vi "test_PhotonPoseEstimator_ClosestToRefPose.vi"(8 "error in (no error)":errorcluster) -> (0 "error out":errorcluster, 3 "Test Passed":bool)   [LabVIEW 2019]
uses:
  <vilib>/Rock Robotics/WPI/ThirdParty/PhotonVisionLib/TypeDef/PhotonEstimatedRobotPoseType.ctl
  <vilib>/Rock Robotics/WPI/ThirdParty/JAS_Junk/TrajLib/TypeDef/POSE3D.ctl
  <vilib>/Rock Robotics/WPI/ThirdParty/JAS_Junk/TrajLib/TypeDef/TRANSLATION3D.ctl
  <vilib>/Rock Robotics/WPI/ThirdParty/JAS_Junk/TrajLib/TypeDef/ROTATION3D.ctl
  <vilib>/Rock Robotics/WPI/ThirdParty/JAS_Junk/TrajLib/TypeDef/QUATERNION.ctl
  <vilib>/Rock Robotics/WPI/ThirdParty/PhotonVisionLib/TypeDef/PhotonTrackedTargetType.ctl
  <vilib>/Rock Robotics/WPI/ThirdParty/PhotonVisionLib/TypeDef/TargetCornerType.ctl
  <vilib>/Rock Robotics/WPI/ThirdParty/JAS_Junk/TrajLib/TypeDef/TRANSFORM3D.ctl
  <vilib>/Rock Robotics/WPI/ThirdParty/PhotonPoseStrategy_ENUM.ctl
  <vilib>/Rock Robotics/WPI/ThirdParty/JAS_Junk/TrajLib/VI/Quaternion_New.vi
  <vilib>/Rock Robotics/WPI/ThirdParty/PhotonVisionLib/SubVI/PhotonTargetModel_New_AprilTag16h5.vi
  <vilib>/Rock Robotics/WPI/ThirdParty/PhotonVisionLib/SubVI/PhotonPoseEstimator_Update_All.vi
  <vilib>/Rock Robotics/WPI/ThirdParty/PhotonVisionLib/SubVI/PhotonTargetModel_New_RectPlanar.vi
  <vilib>/Rock Robotics/WPI/ThirdParty/JAS_Junk/TrajLib/Conv_Inches_Meters.vi
  <vilib>/Rock Robotics/WPI/ThirdParty/PhotonVisionLib/SubVI/PhotonPoseEstimator_SetLastPose.vi
  <vilib>/Rock Robotics/WPI/ThirdParty/PhotonVisionLib/SubVI/PhotonPoseEstimator_GetEmptyPose.vi
  <vilib>/Rock Robotics/WPI/ThirdParty/PhotonVisionLib/SubVI/PhotonPoseEstimator_lowestAmbiguityStrategy.vi
  <vilib>/Rock Robotics/WPI/ThirdParty/PhotonVisionLib/SubVI/PhotonPoseEstimator_closestToCameraHeightStrategy.vi
  <vilib>/Rock Robotics/WPI/ThirdParty/PhotonVisionLib/SubVI/PhotonPoseEstimator_closestToReferencePoseStrategy.vi
  <vilib>/Rock Robotics/WPI/ThirdParty/PhotonVisionLib/SubVI/PhotonPoseEstimator_GetReferencePose.vi
  <vilib>/Rock Robotics/WPI/ThirdParty/PhotonVisionLib/SubVI/PhotonPoseEstimator_GetLastPose.vi
  <vilib>/Rock Robotics/WPI/ThirdParty/PhotonVisionLib/SubVI/PhotonPoseEstimator_averageBestTargetsStrategy.vi
  <vilib>/Rock Robotics/WPI/ThirdParty/PhotonVisionLib/SubVI/PhotonPoseEstimator_multiTagOnCoprocStrategy.vi
  <vilib>/Rock Robotics/WPI/ThirdParty/PhotonVisionLib/SubVI/PhotonTargetModel_New.vi
  <vilib>/Rock Robotics/WPI/ThirdParty/JAS_Junk/TrajLib/VI/Rotation3d_Create_AxisAngle.vi
  <vilib>/Rock Robotics/WPI/ThirdParty/JAS_Junk/TrajLib/VI/Pose3d_New.vi
  <vilib>/Rock Robotics/WPI/ThirdParty/PhotonVisionLib/SubVI/PhotonPipelineResult_HasTargets.vi
  <vilib>/Rock Robotics/WPI/ThirdParty/PhotonVisionLib/SubVI/PhotonPipelineResult_GetTargets.vi
  <vilib>/Rock Robotics/WPI/ThirdParty/PhotonVisionLib/SubVI/PhotonTrackedTarget_GetPoseAmbiguity.vi
  <vilib>/Rock Robotics/WPI/ThirdParty/PhotonVisionLib/SubVI/PhotonTrackedTarget_GetFiducialId.vi
  <vilib>/Rock Robotics/WPI/ThirdParty/PhotonVisionLib/SubVI/PhotonPoseEstimator_GetFieldTags.vi
  <vilib>/Rock Robotics/WPI/ThirdParty/JAS_Junk/TrajLib/VI/AprilTagFieldLayout_GetTagPose.vi
  <vilib>/Rock Robotics/WPI/ThirdParty/JAS_Junk/TrajLib/VI/Pose3d_TransformBy.vi
  <vilib>/Rock Robotics/WPI/ThirdParty/PhotonVisionLib/SubVI/PhotonTrackedTarget_GetBestCameraToTarget.vi
  <vilib>/Rock Robotics/WPI/ThirdParty/JAS_Junk/TrajLib/VI/Transform3d_Inverse.vi
  <vilib>/Rock Robotics/WPI/ThirdParty/PhotonVisionLib/SubVI/PhotonPoseEstimator_GetHighestAmbiguity.vi
  <vilib>/Rock Robotics/WPI/ThirdParty/PhotonVisionLib/SubVI/PhotonPipelineResult_GetTimeStampSecs.vi
  <vilib>/Rock Robotics/WPI/ThirdParty/PhotonVisionLib/SubVI/PhotonPoseEstimator_GetRobotToCameraTransform.vi
  <vilib>/Rock Robotics/WPI/ThirdParty/PhotonVisionLib/SubVI/PhotonEstimatedRobotPose_New.vi
  <vilib>/Rock Robotics/WPI/ThirdParty/PhotonVisionLib/SubVI/PhotonPoseEstimator_closestToCameraHeightStrategy_calc.vi
  <vilib>/Rock Robotics/WPI/ThirdParty/PhotonVisionLib/SubVI/PhotonTrackedTarget_GetAltCameraToTarget.vi
  <vilib>/Rock Robotics/WPI/ThirdParty/PhotonVisionLib/SubVI/PhotonPoseEstimator_closestToReferencePoseStrategy_calc.vi
  <vilib>/Rock Robotics/WPI/ThirdParty/PhotonVisionLib/SubVI/PhotonPoseEstimator_averageBestTargetsStrategy_calc.vi
  <vilib>/Rock Robotics/WPI/ThirdParty/JAS_Junk/TrajLib/VI/Rotation3d_Plus.vi
  <vilib>/Rock Robotics/WPI/ThirdParty/JAS_Junk/TrajLib/VI/Translation3d_Plus.vi
  <vilib>/Rock Robotics/WPI/ThirdParty/JAS_Junk/TrajLib/VI/Translation3d_Times.vi
  <vilib>/Rock Robotics/WPI/ThirdParty/JAS_Junk/TrajLib/VI/Rotation3d_Times.vi
  <vilib>/Rock Robotics/WPI/ThirdParty/JAS_Junk/TrajLib/VI/Rotation3d_Create_Default.vi
  <vilib>/Rock Robotics/WPI/ThirdParty/JAS_Junk/TrajLib/VI/Translation3d_Create_Default.vi
  <vilib>/Rock Robotics/WPI/ThirdParty/JAS_Junk/TrajLib/VI/Pose3d_New_Default.vi
  <vilib>/Rock Robotics/WPI/ThirdParty/JAS_Junk/TrajLib/VI/Pose3d_Plus.vi
  <vilib>/Rock Robotics/WPI/ThirdParty/JAS_Junk/TrajLib/VI/Pose3d_RelativeTo.vi
  <vilib>/Rock Robotics/WPI/ThirdParty/JAS_Junk/TrajLib/VI/AprilTagFieldLayout_GetOriginPosition.vi
  <vilib>/Rock Robotics/WPI/ThirdParty/PhotonVisionLib/SubVI/PhotonPipelineResult_GetMultiTagResult.vi
  <vilib>/Rock Robotics/WPI/ThirdParty/JAS_Junk/TrajLib/VI/Vector_Norm.vi
  <vilib>/Rock Robotics/WPI/ThirdParty/JAS_Junk/TrajLib/VecBuilder_ArrayBy1Fill.vi
  <vilib>/Rock Robotics/WPI/ThirdParty/JAS_Junk/TrajLib/VI/AprilTag_GetAll.vi
  <vilib>/Rock Robotics/WPI/ThirdParty/JAS_Junk/TrajLib/VI/Pose3d_getTranslation3d.vi
  <vilib>/Rock Robotics/WPI/ThirdParty/JAS_Junk/TrajLib/VI/Pose3d_getRotation3d.vi
  <vilib>/Rock Robotics/WPI/ThirdParty/JAS_Junk/TrajLib/VI/Transform3d_GetTranslation3d.vi
  <vilib>/Rock Robotics/WPI/ThirdParty/JAS_Junk/TrajLib/VI/Transform3d_GetRotation3d.vi
  <vilib>/Rock Robotics/WPI/ThirdParty/JAS_Junk/TrajLib/VI/Translation3d_RotateBy.vi
  <vilib>/Rock Robotics/WPI/ThirdParty/JAS_Junk/TrajLib/VI/Translation3d_ToTranslation2d.vi
  <vilib>/Rock Robotics/WPI/ThirdParty/JAS_Junk/TrajLib/VI/Rotation3d_ToRotation2d.vi
  <vilib>/Rock Robotics/WPI/ThirdParty/JAS_Junk/TrajLib/Transform2d_Create_TransRot.vi
  <vilib>/Rock Robotics/WPI/ThirdParty/JAS_Junk/TrajLib/VI/Rotation3d_UnaryMinus.vi
  <vilib>/Rock Robotics/WPI/ThirdParty/JAS_Junk/TrajLib/VI/Translation3d_UnaryMinus.vi
  <vilib>/Rock Robotics/WPI/ThirdParty/JAS_Junk/TrajLib/VI/Transform3d_GetXYZ.vi
  <vilib>/Rock Robotics/WPI/ThirdParty/JAS_Junk/TrajLib/VI/Pose3d_getXYZ.vi
  <vilib>/Rock Robotics/WPI/ThirdParty/PhotonVisionLib/SubVI/PhotonPoseEstimator_CalcDifference.vi
  <vilib>/Rock Robotics/WPI/ThirdParty/JAS_Junk/TrajLib/VI/Rotation3d_RotateBy.vi
  <vilib>/Rock Robotics/WPI/ThirdParty/JAS_Junk/TrajLib/VI/Translation3d_GetXYZ.vi
  <vilib>/Rock Robotics/WPI/ThirdParty/JAS_Junk/TrajLib/VI/Rotation3d_GetQuaterion.vi
  <vilib>/Rock Robotics/WPI/ThirdParty/JAS_Junk/TrajLib/VI/Quaternion_Get_Vect.vi
  <vilib>/Rock Robotics/WPI/ThirdParty/JAS_Junk/TrajLib/VI/Quaternion_Get_W.vi
  <vilib>/Rock Robotics/WPI/ThirdParty/JAS_Junk/TrajLib/VI/Quaternion_New_Default.vi
  <vilib>/Rock Robotics/WPI/ThirdParty/JAS_Junk/TrajLib/VI/Transform3d_Create_Pose3dPose3d.vi
  <vilib>/Rock Robotics/WPI/ThirdParty/JAS_Junk/TrajLib/MatBuilder_Create.vi
  <vilib>/Rock Robotics/WPI/ThirdParty/JAS_Junk/TrajLib/VI/Quaternion_Times.vi
  <vilib>/Rock Robotics/WPI/ThirdParty/JAS_Junk/TrajLib/VI/Quaternion_Inverse.vi
  <vilib>/Rock Robotics/WPI/ThirdParty/JAS_Junk/TrajLib/VI/Quaternion_Get_All.vi
  <vilib>/Rock Robotics/WPI/ThirdParty/JAS_Junk/TrajLib/Translation2d_Create.vi
  <vilib>/Rock Robotics/WPI/ThirdParty/JAS_Junk/TrajLib/Rotation2d_CreateAngle.vi
  <vilib>/Rock Robotics/WPI/ThirdParty/JAS_Junk/TrajLib/VI/Rotation3d_GetXYZ.vi
  <vilib>/Rock Robotics/WPI/ThirdParty/JAS_Junk/TrajLib/VI/Rotation3d_Create_Quaternion.vi
  <vilib>/Rock Robotics/WPI/ThirdParty/JAS_Junk/TrajLib/VI/Translation3d_GetDistance.vi
  <vilib>/Rock Robotics/WPI/ThirdParty/JAS_Junk/TrajLib/VI/Translation3d_Minus.vi
  <vilib>/Rock Robotics/WPI/ThirdParty/JAS_Junk/TrajLib/VI/Rotation3d_Minus.vi
  <vilib>/Rock Robotics/WPI/ThirdParty/JAS_Junk/TrajLib/VI/Quaternion_Normalize.vi
  <vilib>/Rock Robotics/WPI/ThirdParty/PhotonVisionLib/SubVI/PhotonCamera_GetDistCoeffs.vi
  <vilib>/Rock Robotics/WPI/ThirdParty/PhotonVisionLib/SubVI/PhotonCamera_GetCameraMatrix.vi
  <vilib>/Rock Robotics/WPI/ThirdParty/JAS_Junk/TrajLib/Trajectory_Library.lvlib
  <vilib>/Rock Robotics/WPI/ThirdParty/PhotonVisionLib/PhotonVisionLib.lvlib
panel:
  out "Pos Found":bool
  out "PhotonEstimatedRobotPose":T1={"EstimatedPose"={"Translation3d"={"X"=0.0, "Y"=0.0, "Z"=0.0}, "Rotation3d"={"Q_quaternion"={"R"=1.0, "V"=[0.0, 0.0, 0.0]}}}, "TimeStamp_Seconds"=0.0, "targetsUsed"=[], "Strategy"=enum."LOWEST_AMBIGUITY"} {"targetsUsed"."AltCameraToTarget"."TRANSLATION3D"."Z" format="%14.3f"; "targetsUsed"."AltCameraToTarget"."TRANSLATION3D"."Y" format="%14.3f"; "targetsUsed"."AltCameraToTarget"."TRANSLATION3D"."X" format="%14.3f"; "targetsUsed"."BestCameraToTarget"."TRANSLATION3D"."Z" format="%14.3f"; "targetsUsed"."BestCameraToTarget"."TRANSLATION3D"."Y" format="%14.3f"; "targetsUsed"."BestCameraToTarget"."TRANSLATION3D"."X" format="%14.3f"; "EstimatedPose"."Translation3d"."Z" format="%14.3f"; "EstimatedPose"."Translation3d"."Y" format="%14.3f"; "EstimatedPose"."Translation3d"."X" format="%14.3f"}
  out "Test 0 Passed":bool
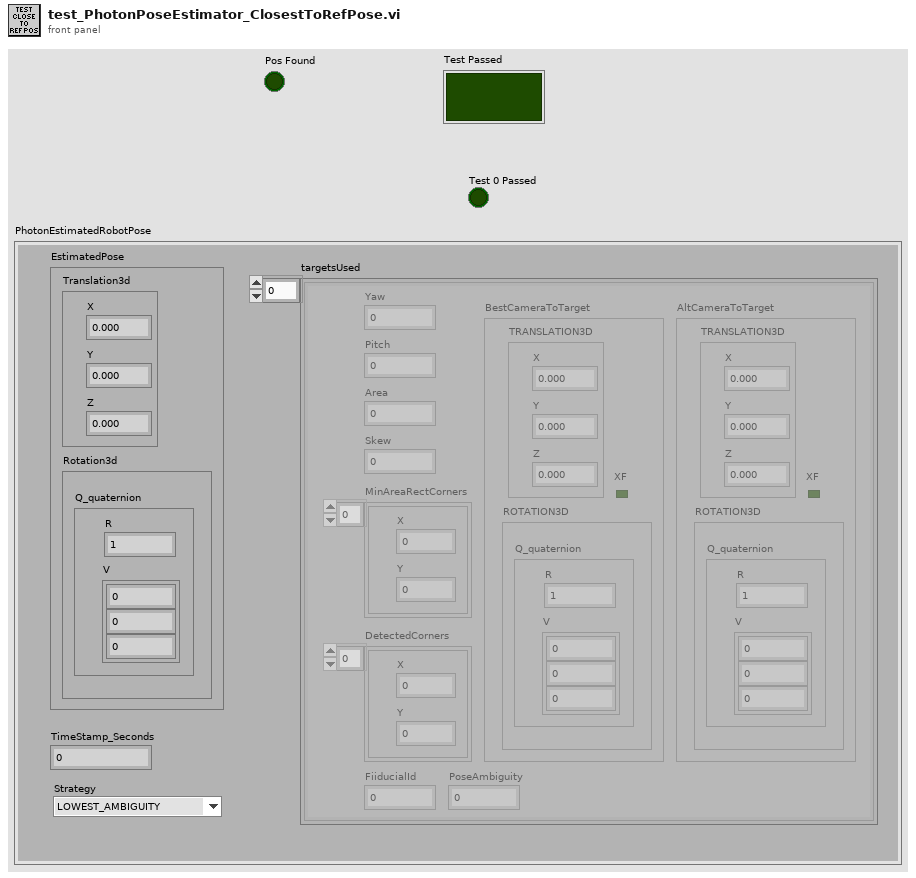
[diagram p1: front panel]
types:
  T1 = typedef "PhotonVisionLib.lvlib/PhotonEstimatedRobotPoseType.ctl" = cluster{"EstimatedPose":T2, "TimeStamp_Seconds":dbl, "targetsUsed":T6[], "Strategy":T9}
  T2 = typedef "Trajectory_Library.lvlib/POSE3D.ctl" = cluster{"Translation3d":T3, "Rotation3d":T4}
  T3 = typedef "Trajectory_Library.lvlib/TRANSLATION3D.ctl" = cluster{"X":dbl, "Y":dbl, "Z":dbl}
  T4 = typedef "Trajectory_Library.lvlib/ROTATION3D.ctl" = cluster{"Q_quaternion":T5}
  T5 = typedef "Trajectory_Library.lvlib/QUATERNION.ctl" = cluster{"R":dbl, "V":dbl[]}
  T6 = typedef "PhotonVisionLib.lvlib/PhotonTrackedTargetType.ctl" = cluster{"Yaw":dbl, "Pitch":dbl, "Area":dbl, "Skew":dbl, "MinAreaRectCorners":T7[], "BestCameraToTarget":T8, "FiiducialId":i32, "AltCameraToTarget":T8, "PoseAmbiguity":dbl, "DetectedCorners":T7[]}
  T7 = typedef "PhotonVisionLib.lvlib/TargetCornerType.ctl" = cluster{"X":dbl, "Y":dbl}
  T8 = typedef "Trajectory_Library.lvlib/TRANSFORM3D.ctl" = cluster{"TRANSLATION3D":T3, "ROTATION3D":T4, "XF":bool}
  T9 = typedef "PhotonVisionLib.lvlib/PhotonPoseStrategy_ENUM.ctl" = enum16{"LOWEST_AMBIGUITY", "CLOSEST_TO_CAMERA_HEIGHT", "CLOSEST_TO_REFERENCE_POSE", "CLOSEST_TO_LAST_POSE", "AVERAGE_BEST_TARGETS", "MULTI_TAG_PNP_ON_COPROCESSOR", "MULTI_TAG_PNP_ON_RIO"}
  T10 = typedef "Trajectory_Library.lvlib/AprilTagFieldLayout.ctl" = cluster{"AprilTagMap":map{i32, T11}, "FieldLength":dbl, "FieldWidth":dbl, "OriginPosition ":T12, "OriginPose3d":T2}
  T11 = typedef "Trajectory_Library.lvlib/AprilTag.ctl" = cluster{"ID":i32, "POSE3D":T2}
  T12 = typedef "Trajectory_Library.lvlib/AprilTagFieldLayoutOrignPosition_ENUM.ctl" = enum16{"kBlueAllianceWallRightSide,", "kRedAllianceWallRightSide,"}
  T13 = typedef "PhotonVisionLib.lvlib/PhotonPipelineResultType.ctl" = cluster{"TargetCount":i32, "Latency_MilliSec":dbl, "Targets":T6[], "TimeStampSec":dbl, "PhotonMultiTargetPNPResult":T14}
  T14 = typedef "PhotonVisionLib.lvlib/PhotonMultiTargetPNPResultType.ctl" = cluster{"PhotonPNPResult":T15, "FiducialIDsUsed":i16[]}
  T15 = typedef "PhotonVisionLib.lvlib/PhotonPNPResultType.ctl" = cluster{"IsPresent":bool, "bestReprojErr":dbl, "altReprojErr":dbl, "ambiguity":dbl, "Best":T8, "Alt":T8}
  T16 = typedef "PhotonVisionLib.lvlib/PhotonPoseEstimatorType.ctl" = cluster{"LastPose":T2, "ReferencePose":T2, "FieldTags":T10, "PrimaryStratety":T9, "Camera":string, "RobotToCamera":T8, "ReportedErrors":dbl[], "HighestAmbiguity":dbl, "MultiTagFallbackStrategy":T9, "PoseCacheTimeoutSec":dbl, "PhotonTargetModel":T17, "BaseNTName":string}
  T17 = typedef "PhotonVisionLib.lvlib/PhotonTargetModel.ctl" = cluster{"Vertices":T3[], "IsPlaner":bool, "IsSpherical":bool}
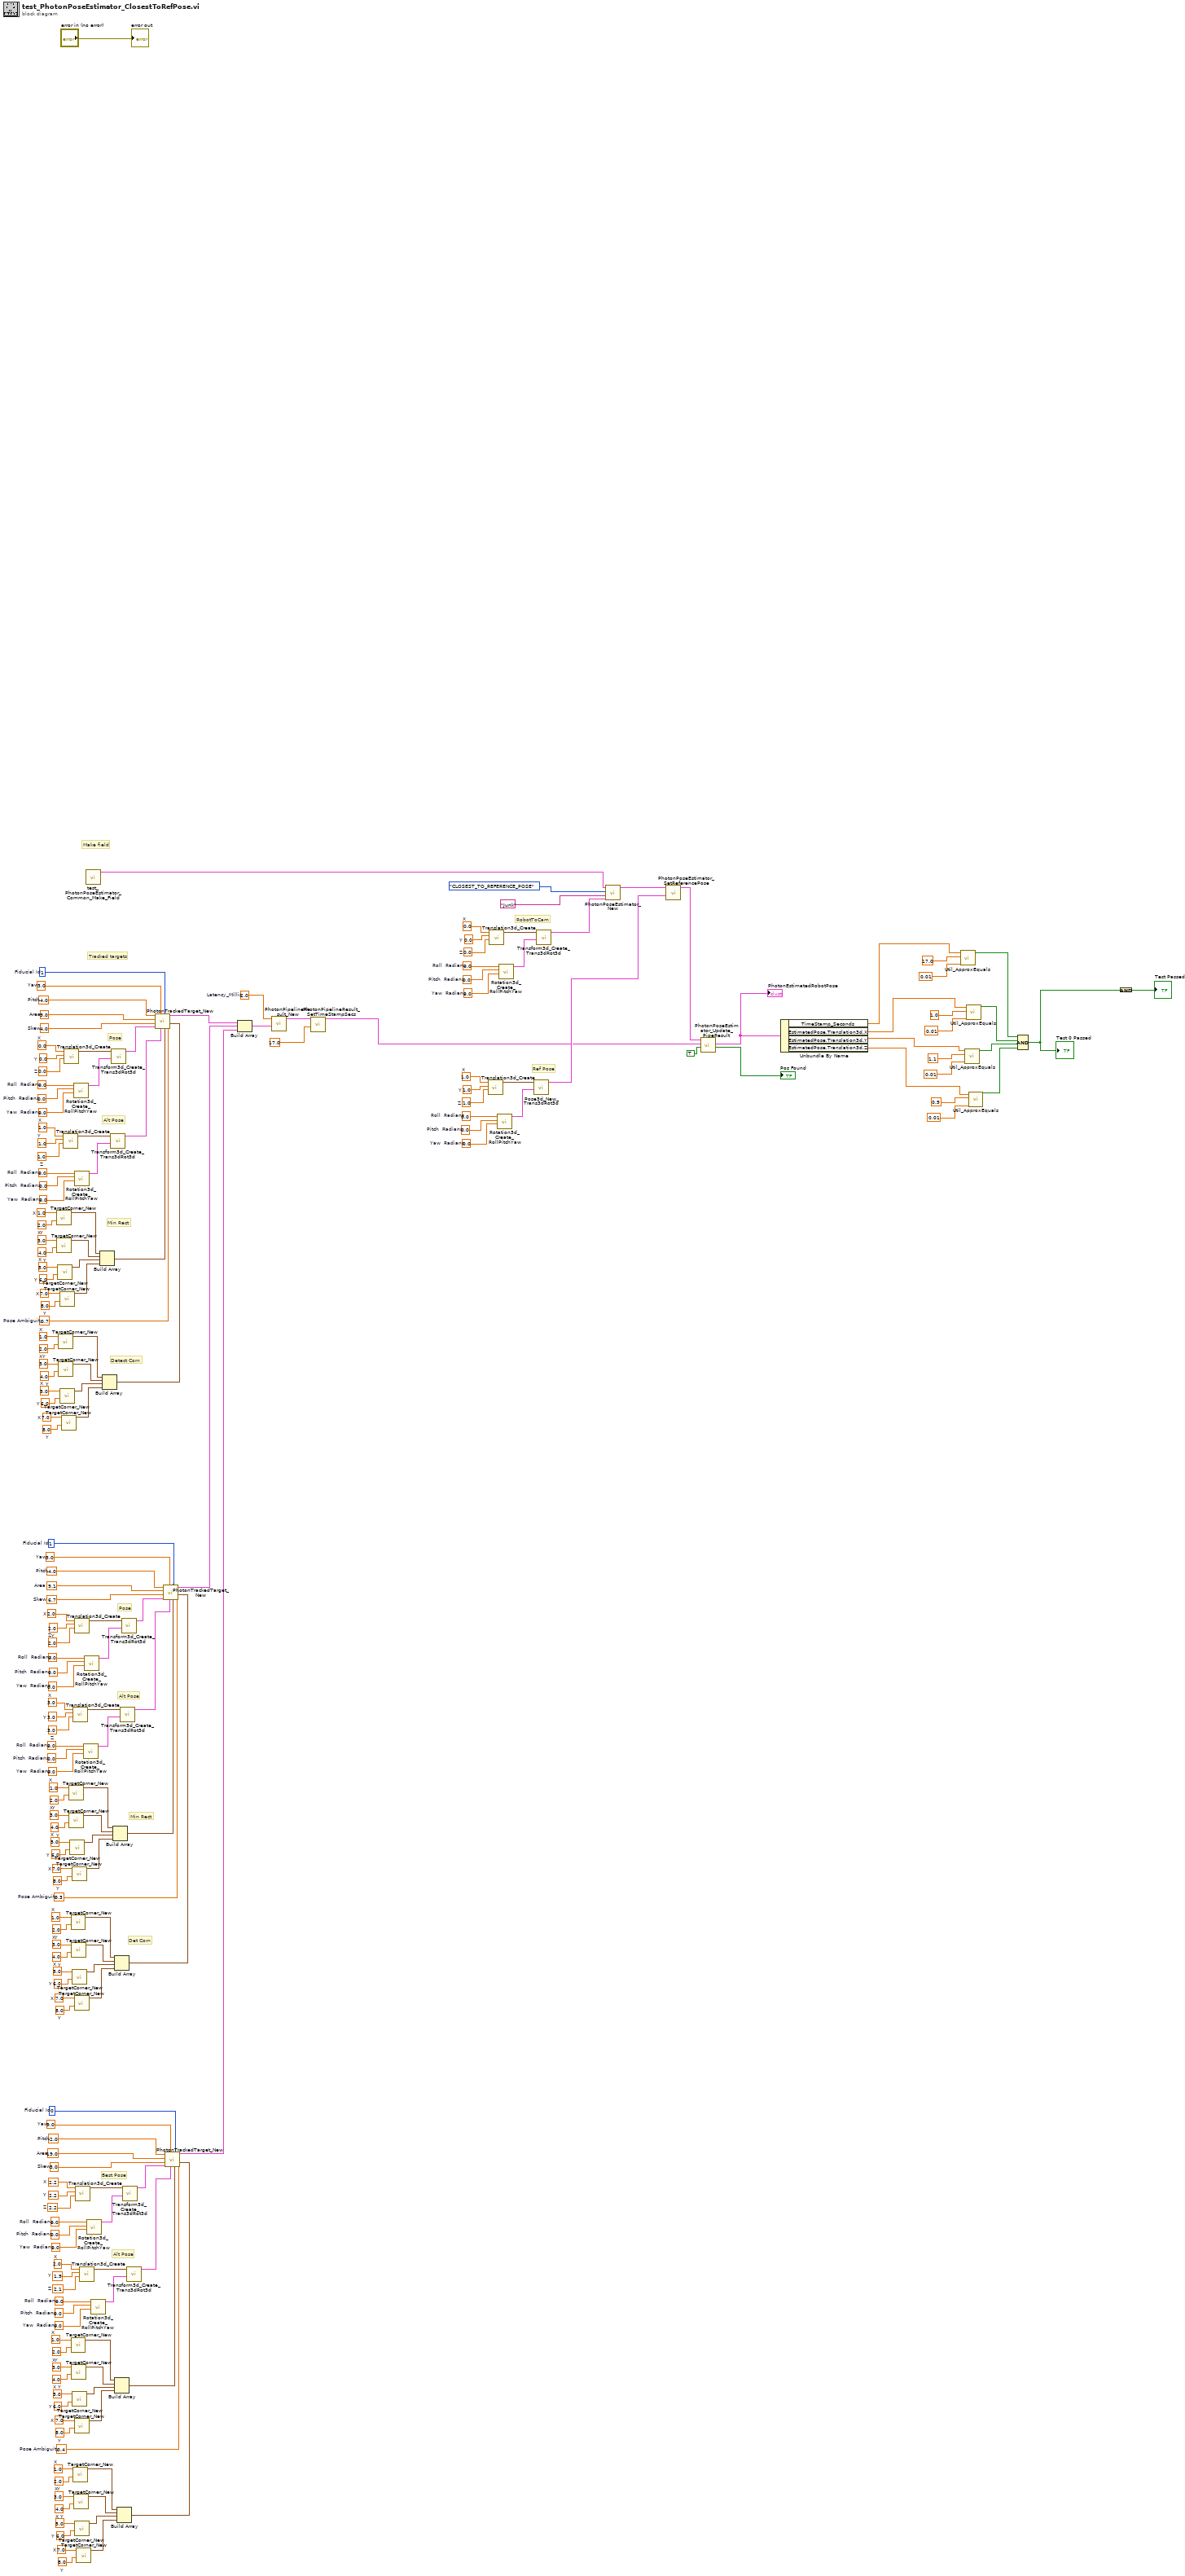
[diagram p0: block diagram]
diagram:
  w11 = 0.0  # Roll  Radians
  w10 = 0.0  # Pitch  Radians
  w9 = 0.0  # Yaw  Radians
  w14 = 1.0  # Z
  w13 = 1.0  # X
  w12 = 1.0  # Y
  w25 = 0.0  # Roll  Radians
  w24 = 0.0  # Pitch  Radians
  w23 = 0.0  # Yaw  Radians
  w28 = 0.0  # Z
  w27 = 0.0  # X
  w26 = 0.0  # Y
  w44 = 2.0  # Latency_Millis
  w54 = 0.0  # Roll  Radians
  w53 = 0.0  # Pitch  Radians
  w52 = 0.0  # Yaw  Radians
  w57 = 2.2  # Z
  w56 = 2.2  # X
  w55 = 2.2  # Y
  w62 = 0.0  # Roll  Radians
  w61 = 0.0  # Pitch  Radians
  w60 = 0.0  # Yaw  Radians
  w65 = 2.1  # Z
  w64 = 2.0  # X
  w63 = 1.9  # Y
  w72 = 7.0  # X
  w73 = 8.0  # Y
  w74 = 5.0  # X
  w75 = 6.0  # Y
  w76 = 3.0  # X
  w77 = 4.0  # Y
  w78 = 1.0  # X
  w79 = 2.0  # Y
  w84 = 7.0  # X
  w85 = 8.0  # Y
  w86 = 5.0  # X
  w87 = 6.0  # Y
  w88 = 3.0  # X
  w89 = 4.0  # Y
  w90 = 1.0  # X
  w91 = 2.0  # Y
  w92 = -2.0  # Pitch
  w93 = 19.0  # Area
  w94 = 3.0  # Skew
  w95 = 0  # Fiducial Id
  w96 = 0.4  # Pose Ambiguity
  w97 = 9.0  # Yaw
  w104 = 0.0  # Roll  Radians
  w103 = 0.0  # Pitch  Radians
  w102 = 0.0  # Yaw  Radians
  w107 = 2.0  # Z
  w106 = 2.0  # X
  w105 = 2.0  # Y
  w112 = 0.0  # Roll  Radians
  w111 = 0.0  # Pitch  Radians
  w110 = 0.0  # Yaw  Radians
  w115 = 3.0  # Z
  w114 = 3.0  # X
  w113 = 3.0  # Y
  w122 = 7.0  # X
  w123 = 8.0  # Y
  w124 = 5.0  # X
  w125 = 6.0  # Y
  w126 = 3.0  # X
  w127 = 4.0  # Y
  w128 = 1.0  # X
  w129 = 2.0  # Y
  w134 = 7.0  # X
  w135 = 8.0  # Y
  w136 = 5.0  # X
  w137 = 6.0  # Y
  w138 = 3.0  # X
  w139 = 4.0  # Y
  w140 = 1.0  # X
  w141 = 2.0  # Y
  w142 = -4.0  # Pitch
  w143 = 9.1  # Area
  w144 = 6.7  # Skew
  w145 = 1  # Fiducial Id
  w146 = 0.3  # Pose Ambiguity
  w147 = 3.0  # Yaw
  w154 = 0.0  # Roll  Radians
  w153 = 0.0  # Pitch  Radians
  w152 = 0.0  # Yaw  Radians
  w157 = 0.0  # Z
  w156 = 0.0  # X
  w155 = 0.0  # Y
  w162 = 0.0  # Roll  Radians
  w161 = 0.0  # Pitch  Radians
  w160 = 0.0  # Yaw  Radians
  w165 = 1.0  # Z
  w164 = 1.0  # X
  w163 = 1.0  # Y
  w172 = 7.0  # X
  w173 = 8.0  # Y
  w174 = 5.0  # X
  w175 = 6.0  # Y
  w176 = 3.0  # X
  w177 = 4.0  # Y
  w178 = 1.0  # X
  w179 = 2.0  # Y
  w184 = 7.0  # X
  w185 = 8.0  # Y
  w186 = 5.0  # X
  w187 = 6.0  # Y
  w188 = 3.0  # X
  w189 = 4.0  # Y
  w190 = 1.0  # X
  w191 = 2.0  # Y
  w192 = -4.0  # Pitch
  w193 = 9.0  # Area
  w194 = 4.0  # Skew
  w195 = 1  # Fiducial Id
  w196 = 0.7  # Pose Ambiguity
  w197 = 3.0  # Yaw
  # "Ref Pose"
  # "RobotToCam"
  # "Det Corn"
  # "Min Rect"
  # "Pose"
  # "Detect Corn"
  # "Min Rect"
  # "Tracked targets"
  # "Make field"
  # "Best Pose"
  # "Alt Pose"
  # "Alt Pose"
  # "Pose"
  # "Alt Pose"
  n1 = call <vilib>:"TargetCorner_New.vi"("Y"=w191, "X"=w190) -> ("TargetCorner"=w183:T7)  [unwired: 9 in]
  n2 = call <vilib>:"TargetCorner_New.vi"("Y"=w189, "X"=w188) -> ("TargetCorner"=w182:T7)  [unwired: 9 in]
  n3 = call <vilib>:"TargetCorner_New.vi"("Y"=w187, "X"=w186) -> ("TargetCorner"=w181:T7)  [unwired: 9 in]
  n4 = call <vilib>:"TargetCorner_New.vi"("Y"=w179, "X"=w178) -> ("TargetCorner"=w171:T7)  [unwired: 9 in]
  n5 = call <vilib>:"TargetCorner_New.vi"("Y"=w177, "X"=w176) -> ("TargetCorner"=w170:T7)  [unwired: 9 in]
  n6 = call <vilib>:"TargetCorner_New.vi"("Y"=w185, "X"=w184) -> ("TargetCorner"=w180:T7)  [unwired: 9 in]
  n7 = call <vilib>:"TargetCorner_New.vi"("Y"=w175, "X"=w174) -> ("TargetCorner"=w169:T7)  [unwired: 9 in]
  n8 = call <vilib>:"TargetCorner_New.vi"("Y"=w173, "X"=w172) -> ("TargetCorner"=w168:T7)  [unwired: 9 in]
  n9 = call <vilib>:"Translation3d_Create.vi"("Z"=w165, "Y"=w163, "X"=w164) -> ("TRANSLATION3D"=w159:T3)  [unwired: 8 in]
  n10 = call <vilib>:"Translation3d_Create.vi"("Z"=w157, "Y"=w155, "X"=w156) -> ("TRANSLATION3D"=w151:T3)  [unwired: 8 in]
  n11 = call <vilib>:"TargetCorner_New.vi"("Y"=w141, "X"=w140) -> ("TargetCorner"=w133:T7)  [unwired: 9 in]
  n12 = call <vilib>:"TargetCorner_New.vi"("Y"=w139, "X"=w138) -> ("TargetCorner"=w132:T7)  [unwired: 9 in]
  n13 = call <vilib>:"TargetCorner_New.vi"("Y"=w137, "X"=w136) -> ("TargetCorner"=w131:T7)  [unwired: 9 in]
  n14 = call <vilib>:"TargetCorner_New.vi"("Y"=w129, "X"=w128) -> ("TargetCorner"=w121:T7)  [unwired: 9 in]
  n15 = call <vilib>:"TargetCorner_New.vi"("Y"=w91, "X"=w90) -> ("TargetCorner"=w83:T7)  [unwired: 9 in]
  n16 = call <vilib>:"TargetCorner_New.vi"("Y"=w127, "X"=w126) -> ("TargetCorner"=w120:T7)  [unwired: 9 in]
  n17 = call <vilib>:"TargetCorner_New.vi"("Y"=w89, "X"=w88) -> ("TargetCorner"=w82:T7)  [unwired: 9 in]
  n18 = call <vilib>:"TargetCorner_New.vi"("Y"=w135, "X"=w134) -> ("TargetCorner"=w130:T7)  [unwired: 9 in]
  n19 = call <vilib>:"TargetCorner_New.vi"("Y"=w125, "X"=w124) -> ("TargetCorner"=w119:T7)  [unwired: 9 in]
  n20 = call <vilib>:"TargetCorner_New.vi"("Y"=w87, "X"=w86) -> ("TargetCorner"=w81:T7)  [unwired: 9 in]
  n21 = call <vilib>:"Translation3d_Create.vi"("Z"=w115, "Y"=w113, "X"=w114) -> ("TRANSLATION3D"=w109:T3)  [unwired: 8 in]
  n22 = call <vilib>:"TargetCorner_New.vi"("Y"=w79, "X"=w78) -> ("TargetCorner"=w71:T7)  [unwired: 9 in]
  n23 = call <vilib>:"Rotation3d_Create_RollPitchYaw.vi"("Yaw"=w152, "Pitch"=w153, "Roll"=w154) -> ("Rotation3d"=w150:T4)  [unwired: 8 in]
  n24 = call <vilib>:"TargetCorner_New.vi"("Y"=w77, "X"=w76) -> ("TargetCorner"=w70:T7)  [unwired: 9 in]
  n25 = call <vilib>:"Rotation3d_Create_RollPitchYaw.vi"("Yaw"=w160, "Pitch"=w161, "Roll"=w162) -> ("Rotation3d"=w158:T4)  [unwired: 8 in]
  n26 = call <vilib>:"Translation3d_Create.vi"("Z"=w107, "Y"=w105, "X"=w106) -> ("TRANSLATION3D"=w101:T3)  [unwired: 8 in]
  n27 = call <vilib>:"TargetCorner_New.vi"("Y"=w123, "X"=w122) -> ("TargetCorner"=w118:T7)  [unwired: 9 in]
  n28 = call <vilib>:"TargetCorner_New.vi"("Y"=w85, "X"=w84) -> ("TargetCorner"=w80:T7)  [unwired: 9 in]
  n29 = call <vilib>:"TargetCorner_New.vi"("Y"=w75, "X"=w74) -> ("TargetCorner"=w69:T7)  [unwired: 9 in]
  n30 = call <vilib>:"Translation3d_Create.vi"("Z"=w57, "Y"=w55, "X"=w56) -> ("TRANSLATION3D"=w51:T3)  [unwired: 8 in]
  n31 = call <vilib>:"TargetCorner_New.vi"("Y"=w73, "X"=w72) -> ("TargetCorner"=w68:T7)  [unwired: 9 in]
  n32 = call <vilib>:"Translation3d_Create.vi"("Z"=w65, "Y"=w63, "X"=w64) -> ("TRANSLATION3D"=w59:T3)  [unwired: 8 in]
  n33 = call <vilib>:"Rotation3d_Create_RollPitchYaw.vi"("Yaw"=w110, "Pitch"=w111, "Roll"=w112) -> ("Rotation3d"=w108:T4)  [unwired: 8 in]
  n34 = call <vilib>:"Rotation3d_Create_RollPitchYaw.vi"("Yaw"=w102, "Pitch"=w103, "Roll"=w104) -> ("Rotation3d"=w100:T4)  [unwired: 8 in]
  n35 = call "test_PhotonPoseEstimator_Common_Make_Field.vi"() -> ("AprilTagFieldLayout"=w40:T10)  [unwired: 11 in]
  n36 = call <vilib>:"Rotation3d_Create_RollPitchYaw.vi"("Yaw"=w52, "Pitch"=w53, "Roll"=w54) -> ("Rotation3d"=w50:T4)  [unwired: 8 in]
  n37 = call <vilib>:"Rotation3d_Create_RollPitchYaw.vi"("Yaw"=w60, "Pitch"=w61, "Roll"=w62) -> ("Rotation3d"=w58:T4)  [unwired: 8 in]
  n38 = Build Array(w183, w182, w181, w180) -> (w167:T7[])
  n39 = Build Array(w171, w170, w169, w168) -> (w166:T7[])
  n40 = call <vilib>:"Transform3d_Create_Trans3dRot3d.vi"("Rotation3d"=w158, "Translation3d"=w159) -> ("Transform3d"=w148:T8)  [unwired: 9 in]
  n41 = call <vilib>:"Transform3d_Create_Trans3dRot3d.vi"("Rotation3d"=w150, "Translation3d"=w151) -> ("Transform3d"=w149:T8)  [unwired: 9 in]
  n42 = Build Array(w133, w132, w131, w130) -> (w117:T7[])
  n43 = Build Array(w121, w120, w119, w118) -> (w116:T7[])
  n44 = Build Array(w83, w82, w81, w80) -> (w67:T7[])
  n45 = Build Array(w71, w70, w69, w68) -> (w66:T7[])
  n46 = call <vilib>:"Transform3d_Create_Trans3dRot3d.vi"("Rotation3d"=w108, "Translation3d"=w109) -> ("Transform3d"=w98:T8)  [unwired: 9 in]
  n47 = call <vilib>:"Transform3d_Create_Trans3dRot3d.vi"("Rotation3d"=w100, "Translation3d"=w101) -> ("Transform3d"=w99:T8)  [unwired: 9 in]
  n48 = call <vilib>:"Transform3d_Create_Trans3dRot3d.vi"("Rotation3d"=w50, "Translation3d"=w51) -> ("Transform3d"=w49:T8)  [unwired: 9 in]
  n49 = call <vilib>:"Transform3d_Create_Trans3dRot3d.vi"("Rotation3d"=w58, "Translation3d"=w59) -> ("Transform3d"=w48:T8)  [unwired: 9 in]
  n50 = call <vilib>:"PhotonTrackedTarget_New.vi"("Pose Ambiguity"=w196, "DetectedCorners"=w166, "MinAreaRectCorners"=w167, "Fiducial Id"=w195, "AltCameraToTarget"=w148, "Yaw"=w197, "BestCameraToTarget"=w149, "Skew"=w194, "Area"=w193, "Pitch"=w192) -> ("TrackedTarget"=w47:T6)  [unwired: 1 in]
  n51 = call <vilib>:"PhotonTrackedTarget_New.vi"("Pose Ambiguity"=w146, "DetectedCorners"=w116, "MinAreaRectCorners"=w117, "Fiducial Id"=w145, "AltCameraToTarget"=w98, "Yaw"=w147, "BestCameraToTarget"=w99, "Skew"=w144, "Area"=w143, "Pitch"=w142) -> ("TrackedTarget"=w46:T6)  [unwired: 1 in]
  n52 = call <vilib>:"PhotonTrackedTarget_New.vi"("Pose Ambiguity"=w96, "DetectedCorners"=w66, "MinAreaRectCorners"=w67, "Fiducial Id"=w95, "AltCameraToTarget"=w48, "Yaw"=w97, "BestCameraToTarget"=w49, "Skew"=w94, "Area"=w93, "Pitch"=w92) -> ("TrackedTarget"=w45:T6)  [unwired: 1 in]
  n53 = Build Array(w47, w46, w45) -> (w43:T6[])
  n54 = call <vilib>:"PhotonPipelineResult_New.vi"("TrackedTargets"=w43, "Latency_Millis"=w44) -> ("PhotonPipelineResult"=w42:T13)  [unwired: 9 in]
  n55 = call <vilib>:"PhotonPipelineResult_SetTimeStampSecs.vi"("TimeStampSec"=17.0, "PhotonPipelineResult"=w42) -> ("Out PhotonPipelineResult"=w3:T13)  [unwired: 9 in]
  n56 = call <vilib>:"Translation3d_Create.vi"("Z"=w14, "Y"=w12, "X"=w13) -> ("TRANSLATION3D"=w8:T3)  [unwired: 8 in]
  n57 = call <vilib>:"Translation3d_Create.vi"("Z"=w28, "Y"=w26, "X"=w27) -> ("TRANSLATION3D"=w22:T3)  [unwired: 8 in]
  n58 = call <vilib>:"Rotation3d_Create_RollPitchYaw.vi"("Yaw"=w9, "Pitch"=w10, "Roll"=w11) -> ("Rotation3d"=w7:T4)  [unwired: 8 in]
  n59 = call <vilib>:"Rotation3d_Create_RollPitchYaw.vi"("Yaw"=w23, "Pitch"=w24, "Roll"=w25) -> ("Rotation3d"=w21:T4)  [unwired: 8 in]
  n60 = call <vilib>:"Pose3d_New_Trans3dRot3d.vi"("Rotation3d"=w7, "Translation3d"=w8) -> ("outPose3d"=w6:T2)  [unwired: 9 in]
  n61 = call <vilib>:"Transform3d_Create_Trans3dRot3d.vi"("Rotation3d"=w21, "Translation3d"=w22) -> ("Transform3d"=w20:T8)  [unwired: 9 in]
  n62 = call <vilib>:"PhotonPoseEstimator_New.vi"("RobotToCamera"=w20, "Camera"="Junk", "Strategy"=PhotonPoseStrategy_ENUM."CLOSEST_TO_REFERENCE_POSE", "AprilTagFieldLayout"=w40) -> ("PhotonPoseEstimator"=w15:T16)  [unwired: 7 in]
  n63 = call <vilib>:"PhotonPoseEstimator_SetReferencePose.vi"("ReferencePose"=w6, "PhotonPoseEstimator"=w15) -> ("out PhotonPoseEstimator"=w4:T16)  [unwired: 9 in]
  n64 = call <vilib>:"PhotonPoseEstimator_Update_PipeResult.vi"("Has Results"=TRUE, "PipelineResult"=w3, "PhotonPoseEstimator"=w4) -> ("Pos Found"=→"Pos Found":bool, "PhotonEstimatedRobotPose"=w2:T1)  [unwired: 6 in, 1 out]
  "PhotonEstimatedRobotPose" <- w2
  n65 = Unbundle By Name(w2) -> ("TimeStamp_Seconds"=w16:dbl, "EstimatedPose.Translation3d.X"=w31:dbl, "EstimatedPose.Translation3d.Y"=w30:dbl, "EstimatedPose.Translation3d.Z"=w29:dbl)
  n66 = call <vilib>:"Util_ApproxEquals.vi"("Tolerance"=0.01, "Value 2"=17.0, "Value 1"=w16) -> ("ApproxEquals"=w17:bool)  [unwired: 8 in]
  n67 = call <vilib>:"Util_ApproxEquals.vi"("Tolerance"=0.01, "Value 2"=1.1, "Value 1"=w30) -> ("ApproxEquals"=w33:bool)  [unwired: 8 in]
  n68 = call <vilib>:"Util_ApproxEquals.vi"("Tolerance"=0.01, "Value 2"=1.0, "Value 1"=w31) -> ("ApproxEquals"=w200:bool)  [unwired: 8 in]
  n69 = call <vilib>:"Util_ApproxEquals.vi"("Tolerance"=0.01, "Value 2"=0.9, "Value 1"=w29) -> ("ApproxEquals"=w32:bool)  [unwired: 8 in]
  n70 = Compound Arithmetic op=AND(w17, w200, w33, w32) -> (w198:bool)
  "Test 0 Passed" <- w198
  n71 = Compound Arithmetic op=AND(w198) -> (→"Test Passed":bool)
  "error out" <- "error in (no error)"
